vi "ControlMotorMove.vi"() -> ()   [LabVIEW 2018]
panel:
  in  "位置":T1(ring)
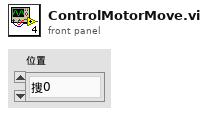
[diagram p1: front panel]
types:
  T1 = enum16{"搜0", "远场相机", "近场相机", "时间波形", "偏振", "能量", "功率", "光谱"}
  T2 = cluster{"电机":enum16{"Z", "Y", "X", "发散角", "俯仰", "旋转"}, "位置":dbl}
  T3 = cluster{"是否停止":enum16{"解除停止", "停止"}, "发生错误停止运行":enum16{"不停止", "停止"}, "发生错误退出运行":enum16{"不退出", "退出"}, "有效电平":cluster{"脉冲信号有效电平":enum16{"低电平有效", "高电平有效"}, "方向信号有效电平 ":enum16{"低电平有效", "高电平有效"}}, "运行脉宽":i32, "编码器使能":enum16{"不使能", "使能"}, "加速度和速度边界":cluster{"加速度最大":i32, "速度最大":i32}, "硬件限位设置":cluster{"正限位使能":enum16{"不使能", "使能"}, "正限位极性":enum16{"低电平有效", "高电平有效"}, "负限位使能 ":enum16{"不使能", "使能"}, "负限位极性 ":enum16{"低电平有效", "高电平有效"}}, "伺服报警":cluster{"伺服报警使能":enum16{"不使能", "使能"}, "伺服报警极性":enum16{"低电平有效", "高电平有效"}}, "电机使能":enum16{"不使能", "使能"}, "输出极性":cluster{"寄存器":u32, " fifo":u32, "Bit":u32, "输出极性控制":enum16{"脉冲+方向", "正负脉冲"}}, "运动模式":enum16{"普通模式", "跟踪模式"}, "加速度 puls/s2":i32, "运动速度":cluster{"峰值速度 puls/s":i32, "起始速度puls/s":i32}, "电机速度归一化常量":dbl}
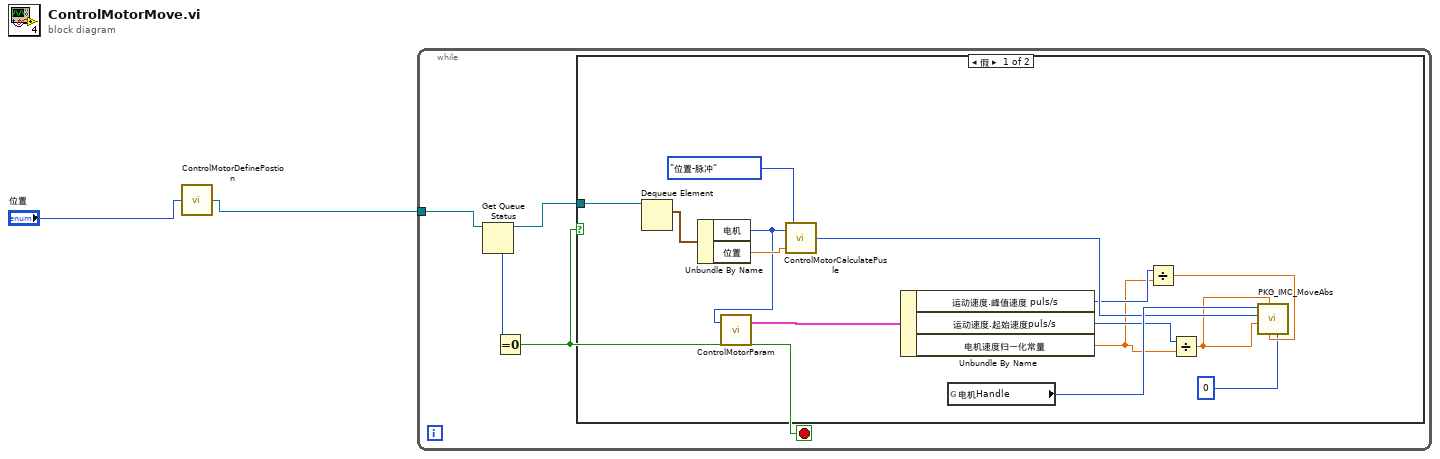
[diagram p0: block diagram]
diagram:
  n1 = call "ControlMotorDefinePostion.vi"("位置"="位置") -> ("位置消息输出"=w1:refnum<queue>)  [unwired: 4 in]
  n2 = while {
    tunnel: w1 -> [w6]
    stop <- w4 stop-if-true
    n3 = Get Queue Status(queue=w6) -> (queue out=w3:refnum<queue>, # elements in queue=w5:i32)  [unwired: 2 in, 6 out]
    n4 = Equal To 0?(x=w5) -> (x = 0?=w4:bool)
    n5 = case shown="假" w4 {
      tunnel: w3 -> [w20 _]
      frame False {
        n6 = Dequeue Element(queue=w20) -> (element=w19:T2)  [unwired: 2 in, 3 out]
        n7 = Unbundle By Name(w19) -> ("电机"=w17:enum16{"Z", "Y", "X", "发散角", "俯仰", "旋转"}, "位置"=w18:dbl)
        n8 = call "ControlMotorParam.vi"("电机"=w17) -> ("轴电机参数输出"=w16:T3)  [unwired: 2 in]
        n9 = call "ControlMotorCalculatePusle.vi"("数据"=w18, "计算状态"=enum32{"位置-脉冲", "脉冲-位置"}."位置-脉冲", "电机"=w17) -> ("dataout"=w14:i32)  [unwired: 2 in]
        n10 = Unbundle By Name(w16) -> ("运动速度.峰值速度 puls/s"=w13:i32, "运动速度.起始速度puls/s"=w11:i32, "电机速度归一化常量"=w10:dbl)
        n11 = global read "参数.vi" "电机Handle"() -> (w15:u32)
        n12 = Divide(x=w13, y=w10) -> (x/y=w12:dbl)
        n13 = Divide(x=w11, y=w10) -> (x/y=w9:dbl)
        n14 = call "PKG_IMC_MoveAbs.vi"("wait"=0, "tgvel"=w12, "endvel"=w9, "startvel"=w9, "pos"=w14, "handle"=w15) -> ()  [unwired: 4 in, 2 out]
      }
      frame True {
      }
    }
  }
